vi "Ignore command if not initialized.vi"(11 "Command in":T1) -> (3 "Command out":T1)   [LabVIEW 2017, in "Magnet module.lvlib"]
doc: "Returns enum with command to ignore message, if module is not initialized. In that case, only \"initialize\" command will be accepted."
uses:
  Magnet module.lvlib
  ctl/Magnet Orders.ctl
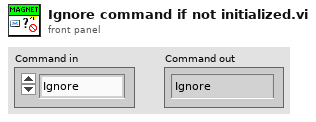
[diagram p1: front panel]
types:
  T1 = typedef "Magnet module.lvlib/Magnet Orders.ctl" = enum16{"Ignore", "Connect", "Update", "Switch mode", "Set field", "Stop ramping", "Equalize output", "Zero output", "Flip polarity", "Blackout", "Set timer", "Eval temperatures", "Disconnect"}
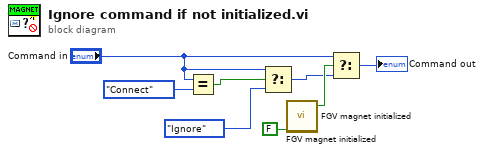
[diagram p0: block diagram]
diagram:
  n1 = Equal?(x="Command in", y=Magnet_Orders."Connect") -> (x = y?=w4:bool)
  n2 = Select(t="Command in", s=w4, f=Magnet_Orders."Ignore") -> (s? t:f=w5:T1)
  n3 = call "FGV magnet initialized.vi"() -> ()  [unwired: 11 in, 1 out]
  n4 = call "FGV magnet initialized.vi"("Write?(F)"=FALSE) -> ("Initialized out"=w7:bool)  [unwired: 10 in]
  n5 = Select(t="Command in", s=w7, f=w5) -> (s? t:f=→"Command out":T1)
